vi "Multi-Graph Facade.vi"(0 "Data In":T4, 2 "Display State In":T2, 3 "Container State":T3) -> (6 "Data Out":T4, 7 "Display State Out":T2, 8 "Action":T1)   [LabVIEW 2009, in "Multi-Graph.xctl"]
doc: "Demonstration of an XControl.\n\nAAL 9/09"
uses:
  Multi-Graph.xctl
  Multi-Graph Data.ctl
  <vilib>/_xctls/Container State.ctl
  Multi-Graph State.ctl
  <vilib>/_xctls/Action.ctl
  <vilib>/measure/maspectr.llb/FFT Power Spectrum for 1 Chan.vi
  <vilib>/_xctls/XControlSupport.lvlib
  <vilib>/measure/NI_MAPro.lvlib
panel:
  out "Waveform Graph":cluster{"f0":dbl, "df":dbl, "magnitude":dbl[]}(graph)
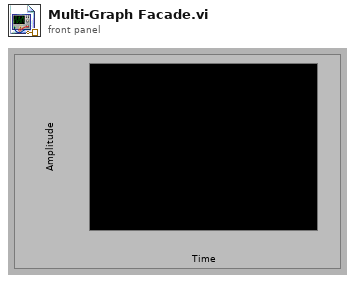
[diagram p1: front panel]
types:
  T1 = typedef "XControlSupport.lvlib/Action.ctl" = cluster{"Data Changed?":bool, "State Changed?":bool, "Action Name":string}
  T2 = typedef "Multi-Graph.xctl/Multi-Graph State.ctl" = cluster{"Domain":enum16{"Time Domain", "Frequency Domain"}, "MenuRef":refnum<k9>}
  T3 = typedef "XControlSupport.lvlib/Container State.ctl" = cluster{"Indicator?":bool, "Run Mode?":bool, " Refnum":refnum<vi>}
  T4 = typedef "Multi-Graph.xctl/Multi-Graph Data.ctl" = waveform(dbl)
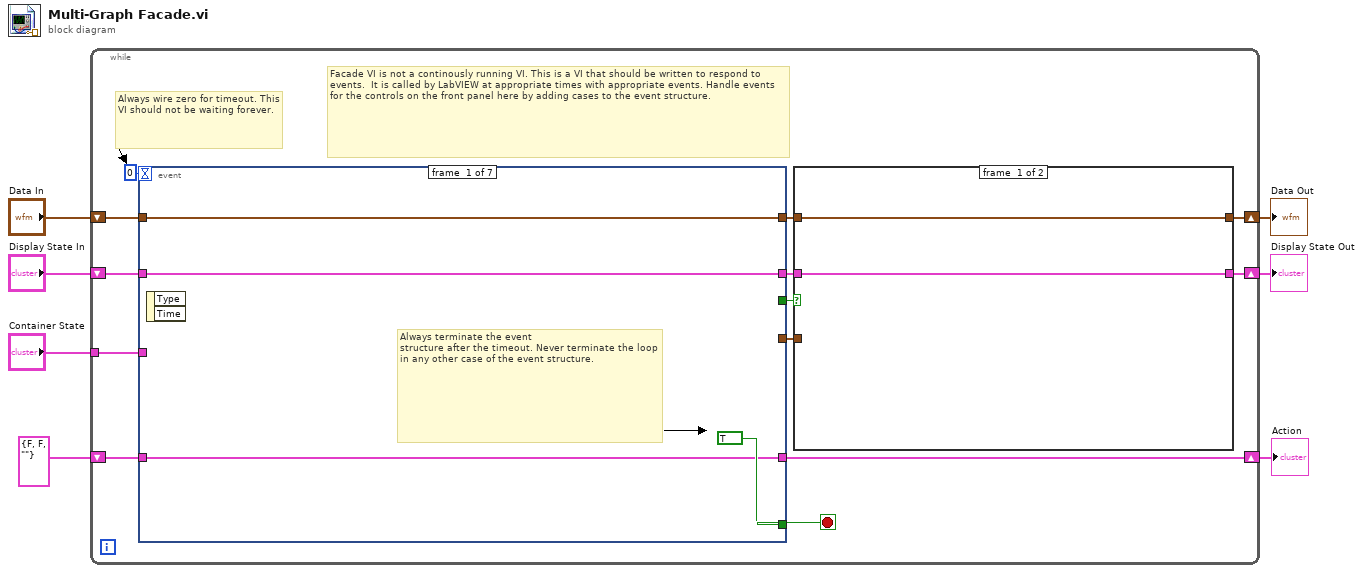
[diagram p0: block diagram]
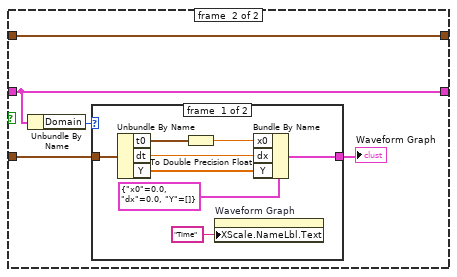
[diagram p2: hidden frame]
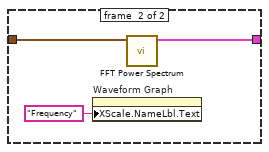
[diagram p3: hidden frame]
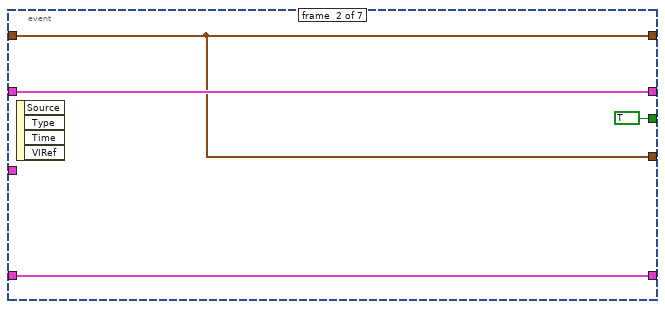
[diagram p4: hidden frame]
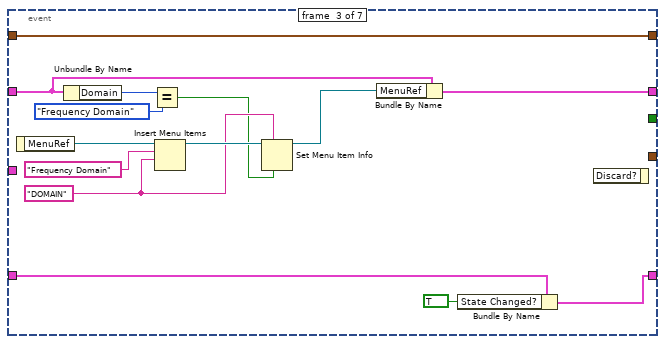
[diagram p5: hidden frame]
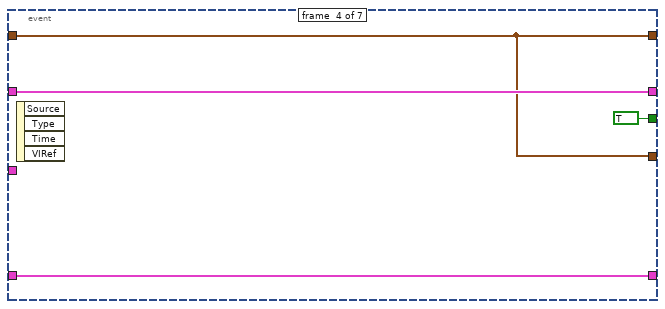
[diagram p6: hidden frame]
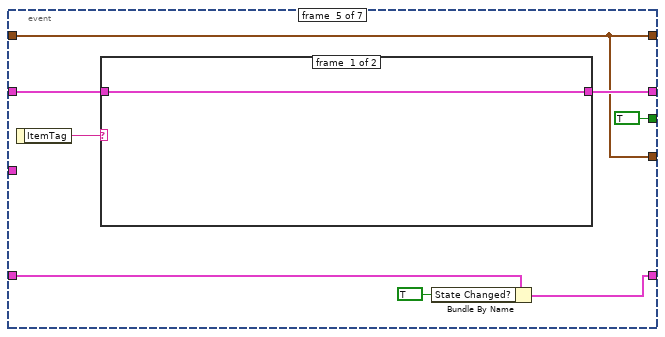
[diagram p7: hidden frame]
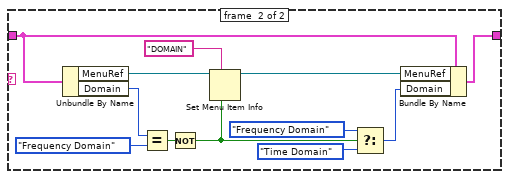
[diagram p8: hidden frame]
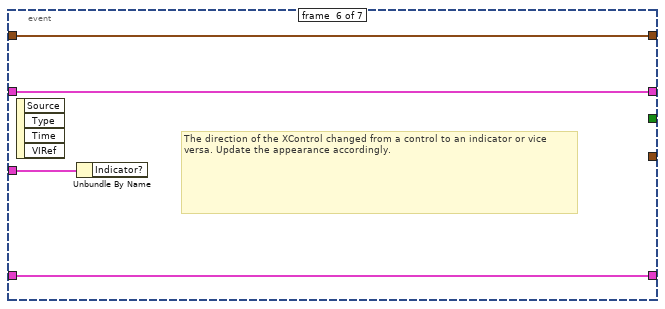
[diagram p9: hidden frame]
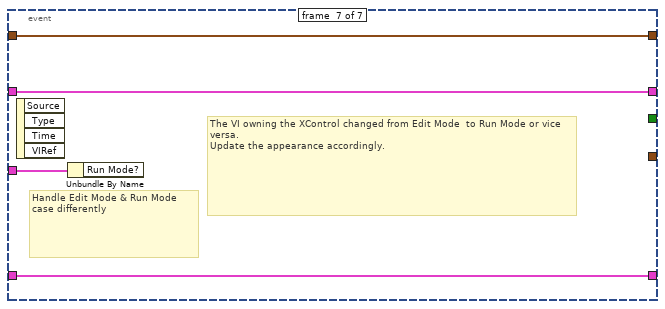
[diagram p10: hidden frame]
diagram:
  n1 = while {
    shift-right: [w8] -> w4
    shift-left: "Display State In" -> [w20]
    tunnel: "Container State" -> [w17]
    shift-right: [w10] -> w7
    shift-left: "Data In" -> [w16]
    shift-right: [w14] -> w2
    shift-left: T1 {"Data Changed?"=FALSE, "State Changed?"=FALSE, "Action Name"=""} ("Action") -> [w15]
    stop <- w19 stop-if-true
    # "Facade VI is not a continously running VI. This is a VI that should be written to respond to events.  It is called by LabVIEW at appropriate times with appropriate events. Handle events for the controls on the front panel here by adding cases to the event structure."
    # "Always wire zero for timeout. This\nVI should not be waiting forever."
    n2 = event shown="[3] Display State Change" {
      selector: _ -> [_ _ _ _ _ _ _]
      dyn-events: _ -> [_ _ _ _ _ _ _]
      timeout: 0 -> [_ _ _ _ _ _ _]
      tunnel: w20 -> [w40 w45 w58 w63 w71 w88 w92]
      tunnel: [w40 w45 w59 w63 w70 w88 w92] -> w9
      tunnel: [TRUE _ _ _ _ _ _] -> w19
      tunnel: w17 -> [_ _ _ _ _ w89 w93]
      tunnel: w16 -> [w39 w43 w51 w61 w66 w87 w91]
      tunnel: [w39 w43 w51 w61 w66 w87 w91] -> w11
      tunnel: [w41 w46 w48 w64 w67 w86 w90] -> w14
      tunnel: w15 -> [w41 w46 w50 w64 w68 w86 w90]
      tunnel: [_ w43 _ w61 w66 _ _] -> w13
      tunnel: [_ TRUE _ TRUE TRUE _ _] -> w12
      event #0 {
        # "Always terminate the event\nstructure after the timeout. Never terminate the loop in any other case of the event structure."
        n3 = event-data() -> ()  [unwired: 1 in, 2 out]
      }
      event #1 {
        n4 = event-data() -> ()  [unwired: 1 in, 4 out]
      }
      event #2 {
        w55 = "DOMAIN"
        n5 = event-data() -> ("MenuRef"=w60:refnum<k9>)  [unwired: 1 in]
        n6 = Unbundle By Name(w58) -> ("Domain"=w54:enum16{"Time Domain", "Frequency Domain"})
        n7 = Equal?(x=w54, y=enum16{"Time Domain", "Frequency Domain"}."Frequency Domain") -> (x = y?=w47:bool)
        n8 = Insert Menu Items(7:w55, 8:"Frequency Domain" ("item names"), 9:w60) -> (3:w56:refnum<k9>)  [unwired: 3 in, 2 out]
        n9 = Set Menu Item Info(6:w47, 7:w55, 11:w56) -> (3:w52:refnum<k9>)  [unwired: 4 in, 1 out]
        n10 = Bundle By Name(cluster=w58, "MenuRef"=w52) -> (w59:T2)
        n11 = Bundle By Name(cluster=w50, "State Changed?"=TRUE) -> (w48:T1)
        n12 = event-data() -> ()  [unwired: 2 in, 1 out]
      }
      event #3 {
        n13 = event-data() -> ()  [unwired: 1 in, 4 out]
      }
      event #4 {
        n14 = event-data() -> ("ItemTag"=w72:string)  [unwired: 1 in]
        n15 = case shown="\"DOMAIN\"" w72 {
          tunnel: w71 -> [w73 w85]
          tunnel: [w73 w84] -> w70
          frame #0 {
          }
          frame #1 {
            n16 = Unbundle By Name(w85) -> ("MenuRef"=w83:refnum<k9>, "Domain"=w81:enum16{"Time Domain", "Frequency Domain"})
            n17 = Equal?(x=w81, y=enum16{"Time Domain", "Frequency Domain"}."Frequency Domain") -> (x = y?=w78:bool)
            n18 = Not(x=w78) -> (.not. x?=w77:bool)
            n19 = Set Menu Item Info(6:w77, 7:"DOMAIN", 11:w83) -> (3:w79:refnum<k9>)  [unwired: 4 in, 1 out]
            n20 = Select(t=enum16{"Time Domain", "Frequency Domain"}."Frequency Domain", s=w77, f=enum16{"Time Domain", "Frequency Domain"}."Time Domain" ("y")) -> (s? t:f=w74:enum16{"Time Domain", "Frequency Domain"})
            n21 = Bundle By Name(cluster=w85, "MenuRef"=w79, "Domain"=w74) -> (w84:T2)
          }
        }
        n22 = Bundle By Name(cluster=w68, "State Changed?"=TRUE) -> (w67:T1)
      }
      event #5 {
        # "The direction of the XControl changed from a control to an indicator or vice versa. Update the appearance accordingly."
        n23 = event-data() -> ()  [unwired: 1 in, 4 out]
        n24 = Unbundle By Name(w89) -> ()  [unwired: 1 out]
      }
      event #6 {
        # "The VI owning the XControl changed from Edit Mode  to Run Mode or vice versa.\nUpdate the appearance accordingly."
        # "Handle Edit Mode & Run Mode\ncase differently"
        n25 = event-data() -> ()  [unwired: 1 in, 4 out]
        n26 = Unbundle By Name(w93) -> ()  [unwired: 1 out]
      }
    }
    n27 = case shown="False" w12 {
      tunnel: w13 -> [_ w25]
      tunnel: [w21 w27] -> w10
      tunnel: w11 -> [w21 w27]
      tunnel: [w22 w23] -> w8
      tunnel: w9 -> [w22 w23]
      frame #0 {
      }
      frame #1 {
        n28 = Unbundle By Name(w23) -> ("Domain"=w26:enum16{"Time Domain", "Frequency Domain"})
        n29 = case shown="\"Frequency Domain\"" w26 {
          tunnel: w25 -> [w33 w38]
          tunnel: [w34 w37] -> w24
          frame #0 {
            n30 = Unbundle By Name(w33) -> ("t0"=w32:timestamp, "dt"=w30:dbl, "Y"=w29:dbl[])
            n31 = To Double Precision Float(number=w32) -> (double precision float=w31:dbl)
            n32 = property on="Waveform Graph" class="WFGraph (strict)"("XScale.NameLbl.Text"="Time" ("X Scale.Name Label.Text")) -> ()  [unwired: 2 in, 2 out]
            n33 = Bundle By Name(cluster=cluster{"x0":dbl, "dx":dbl, "Y":dbl[]} {"x0"=0.0, "dx"=0.0, "Y"=[]} ("power spectrum"), "x0"=w31, "dx"=w30, "Y"=w29) -> (w34:cluster{"x0":dbl, "dx":dbl, "Y":dbl[]})
          }
          frame #1 {
            n34 = property on="Waveform Graph" class="WFGraph (strict)"("XScale.NameLbl.Text"="Frequency" ("X Scale.Name Label.Text")) -> ()  [unwired: 2 in, 2 out]
            n35 = call-poly <vilib>:"FFT Power Spectrum.vi"("time signal"=w38) -> ("power spectrum"=w37:cluster{"f0":dbl, "df":dbl, "magnitude":dbl[]})  [unwired: 7 in, 3 out]
          }
        }
        "Waveform Graph" <- w24
      }
    }
  }
  "Display State Out" <- w4
  "Data Out" <- w7
  "Action" <- w2
